vi "_MobileTest_Publish.vi"(8 "Data":variant) -> ()   [LabVIEW 2019]
uses:
  Public/Documents/National Instruments/TestStand 2019 (64-bit)/Examples/Demos/Mobile Device Test/LabVIEW/Source/Support/Wifi Test Modes.ctl
panel:
  in  "id":u32
  out "data string":string
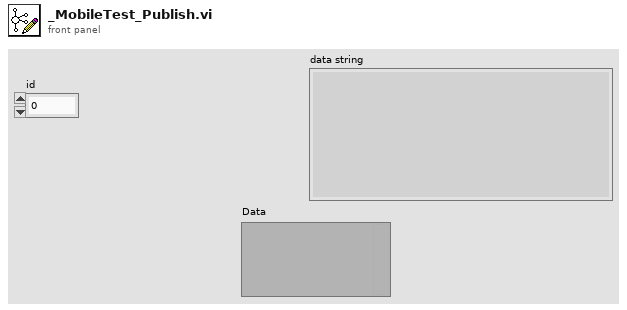
[diagram p1: front panel]
types:
  T1 = typedef "Wifi Test Modes.ctl" = enum16{"802.11b/g/n (QAM-16)", "LTE (QAM-64)", "802.11ac (QAM-256)"}
  T2 = cluster{"QAM Data":cluster{dbl[], dbl[]}, "QAM Data Out":cluster{dbl[], dbl[]}, "symbol map 16 QAM":cdb[], "Mode":T1}
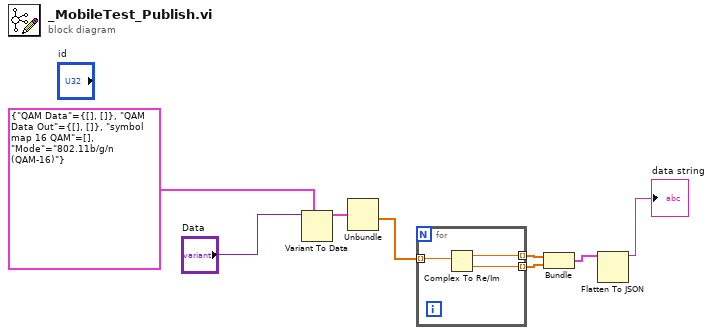
[diagram p0: block diagram]
diagram:
  n1 = Variant To Data(type=T2 {"QAM Data"={[], []}, "QAM Data Out"={[], []}, "symbol map 16 QAM"=[], "Mode"=enum."802.11b/g/n (QAM-16)"} ("output cluster"), Variant="Data") -> (data=w6:T2)  [unwired: 1 in, 1 out]
  n2 = Unbundle(w6) -> ("symbol map 16 QAM"=w5:cdb[])  [unwired: 3 out]
  n3 = for {
    tunnel: w5 -> [w11] mode=indexing
    tunnel: [w10] -> w4 mode=indexing
    tunnel: [w9] -> w3 mode=indexing
    n4 = Complex To Re/Im(x + iy=w11) -> (x=w10:dbl, y=w9:dbl)
  }
  n5 = Bundle(w4, w3) -> (w2:cluster{dbl[], dbl[]})  [unwired: 1 in]
  n6 = Flatten To JSON(anything=w2) -> (JSON string=→"data string":string)  [unwired: 2 in, 1 out]
